vi "PointGrey Grasshopper_Cam.vi"(4 "Frames in sequence":u32, 6 "Image in":variant, 7 "Camera-specific in":variant, 8 "Save path":path, 9 "Capture mode":enum16{"Single frame", "Sequence"}(ring), 10 "Exposure time (s)":dbl, 11 "Operation":T2(ring)) -> (3 "Status":T1, 5 "Camera-specific out":variant)   [LabVIEW 2015]
uses:
  <vilib>/userdefined/High Color/IMAQdx.ctl
  <vilib>/vision/Image Controls.llb/IMAQ Image.ctl
  <vilib>/vision/driver/IMAQdx.llb/IMAQdx Camera Control Mode.ctl
  <vilib>/vision/driver/IMAQdx.llb/IMAQdx Buffer Number Mode.ctl
  <vilib>/vision/driver/NI_Vision_Acquisition_Software.lvlib
  <resource>/objmgr/imaqdx.rc
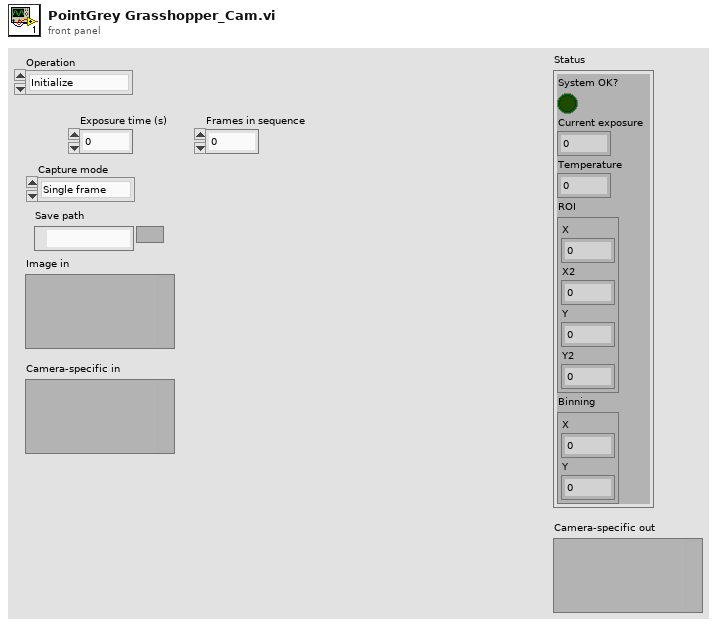
[diagram p1: front panel]
types:
  T1 = cluster{"System OK?":bool, "Current exposure":dbl, "Temperature":dbl, "ROI":cluster{"X":u32, "X2":u32, "Y":u32, "Y2":u32}, "Binning":cluster{"X":u32, "Y":u32}}
  T2 = enum16{"Initialize", "Shut down", "Set capture mode", "Set exposure", "Trigger and read", "Get status", "Other settings"}
  T3 = typedef "IMAQdx.ctl" = refnum<k21>
  T4 = typedef "IMAQ Image.ctl" = refnum<image>
  T5 = cluster{"Frames to capture":u32, "Current camera":i32, "Camera References":T3[], "Camera event refnum":refnum<event-registration>, "Which cameras record":bool[], "Image buffers":T4[]}
  T6 = enum32{"Continuous", "Single frame", "Multi frame"}
  T7 = typedef "NI_Vision_Acquisition_Software.lvlib/IMAQdx Camera Control Mode.ctl" = enum32{"Controller", "Listener"}
  T8 = cluster{"New Image":T4, "Image":refnum<vi>, "FPS target":dbl}
  T9 = enum16{"open", "replace", "create", "open or create", "replace or create", "replace or create with confirmation"}
  T10 = cluster{"File refnum":refnum<file>, "Image File Directory":cluster{cluster{"Field":u16, "Type":u16, "Count":u32, "Value / Offset":u32, "Add IFD Offset?":bool}[], cluster{"Data":u32[], "Add offset?":bool}[]}, "Big endian?":bool, "IFD Offset Size":u32}
  T11 = typedef "NI_Vision_Acquisition_Software.lvlib/IMAQdx Buffer Number Mode.ctl" = enum32{"Next", "Last", "Buffer Number", "Every", "Last New"}
  T12 = cluster{"Type":u32, "Version":u32, "Flags":u32, "SerialNumberHigh":u32, "SerialNumberLow":u32, "BusType":u32, "InterfaceName":string, "VendorName":string, "ModelName":string, "CameraFileName":string, "CameraAttributeURL":string}[]
  T13 = typedef "NI_Vision_Acquisition_Software.lvlib/IMAQdx Attribute Type.ctl" = enum32{"U32", "I64", "DBL", "String", "Enum", "Bool", "Command"}
  T14 = cluster{"Attribute Type":T13, "Readable":bool, "Writable":bool, "Attribute Name":string}[]
  T15 = typedef "Image Type" = u32
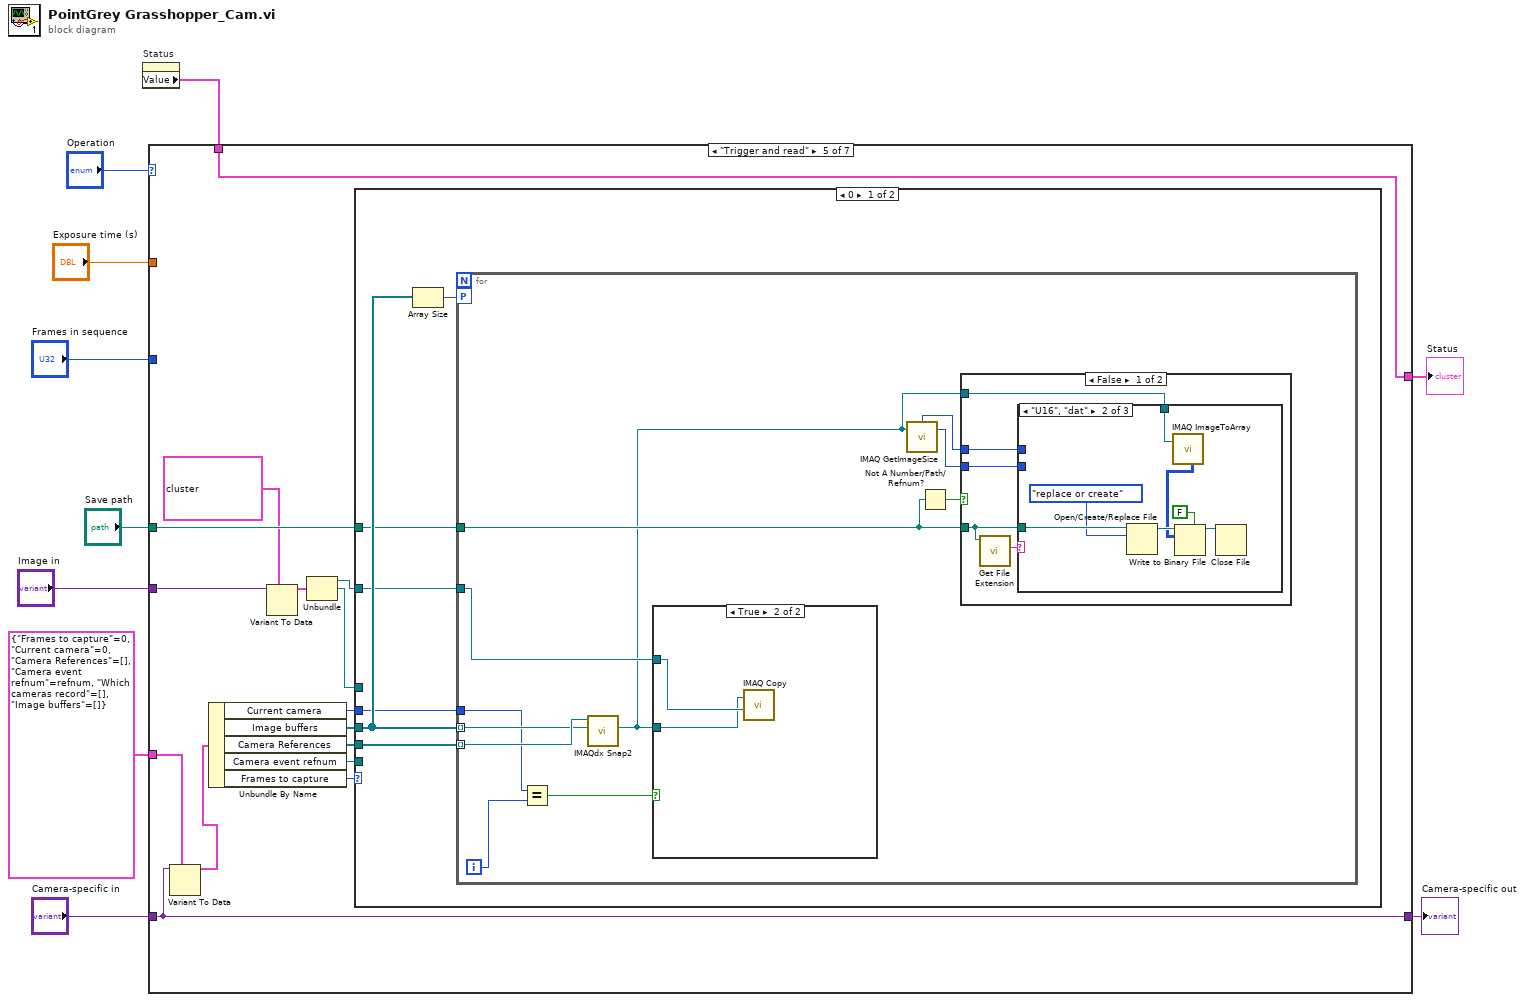
[diagram p0: block diagram]
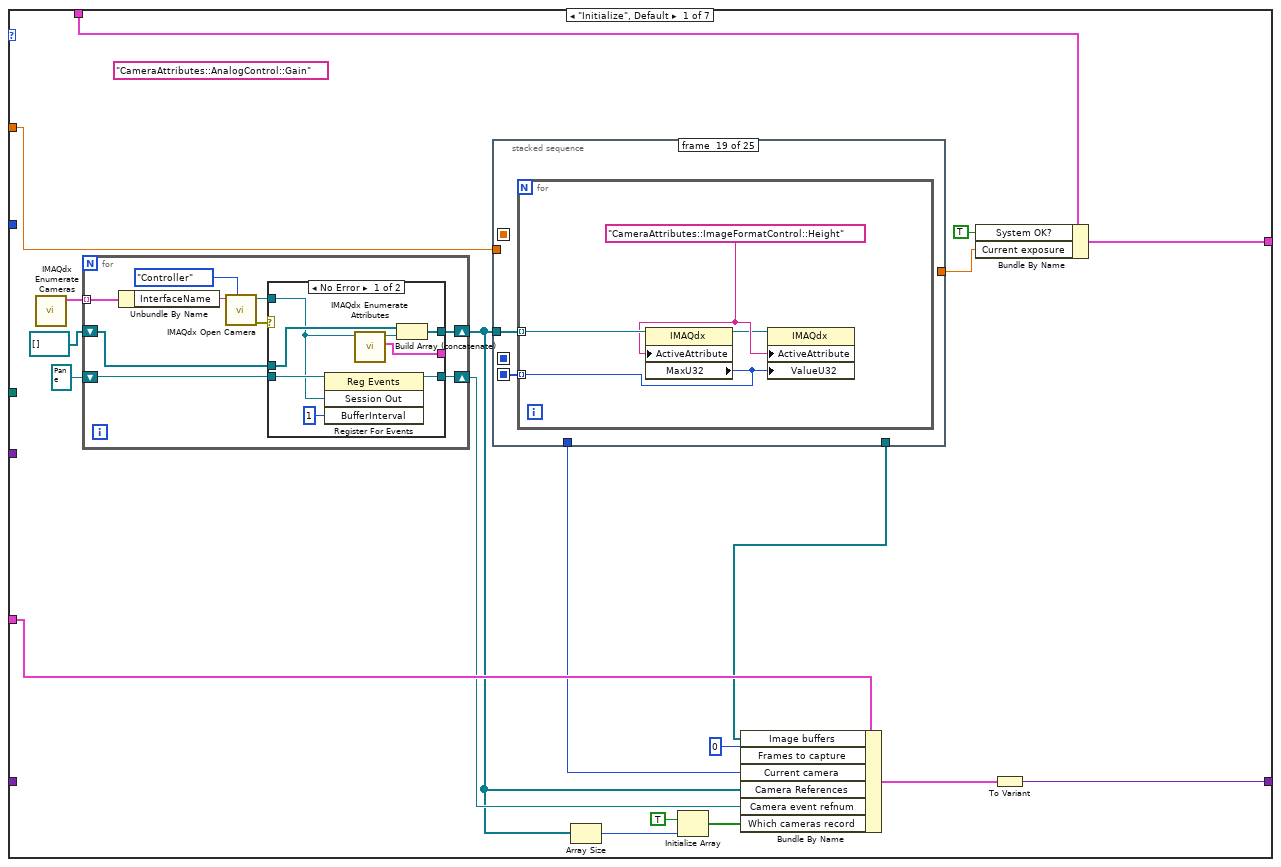
[diagram p2: hidden frame]
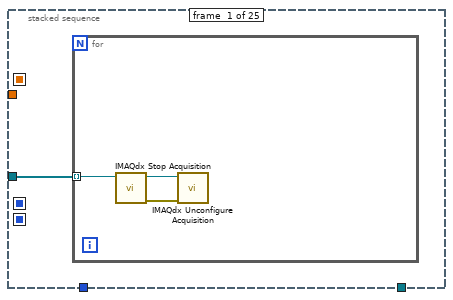
[diagram p3: hidden frame]
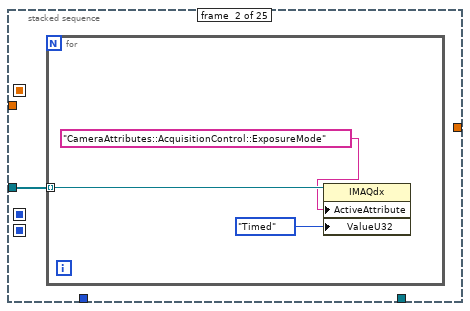
[diagram p4: hidden frame]
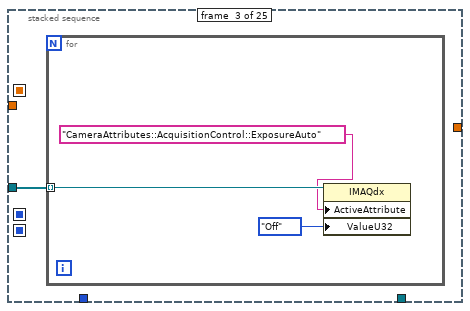
[diagram p5: hidden frame]
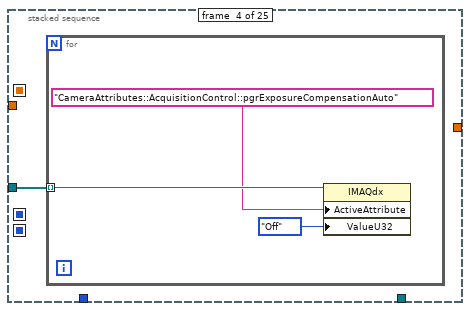
[diagram p6: hidden frame]
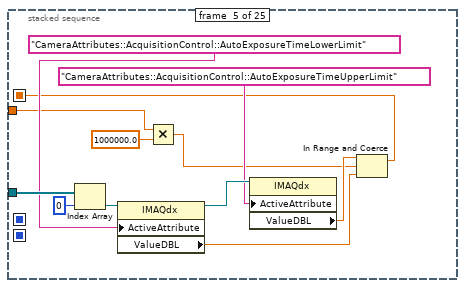
[diagram p7: hidden frame]
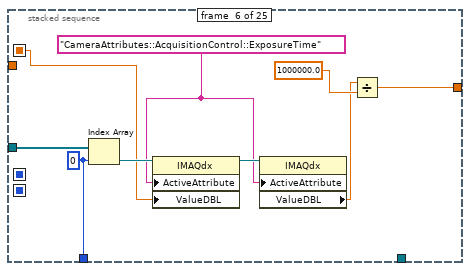
[diagram p8: hidden frame]
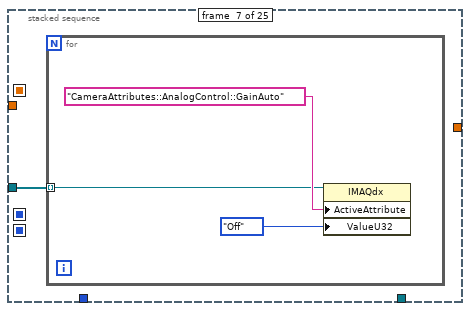
[diagram p9: hidden frame]
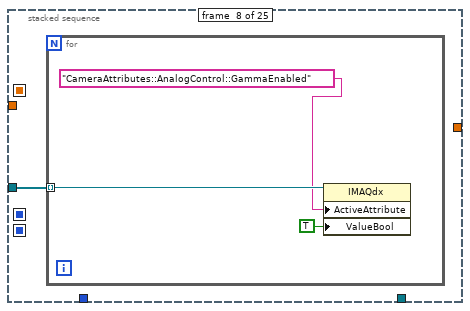
[diagram p10: hidden frame]
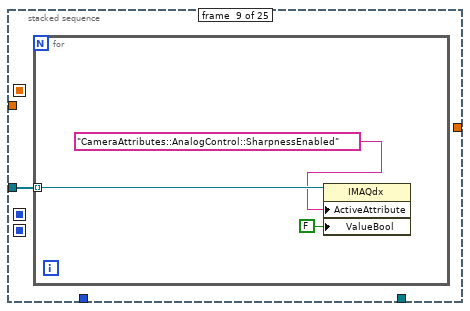
[diagram p11: hidden frame]
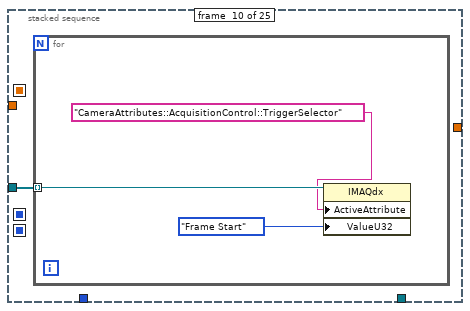
[diagram p12: hidden frame]
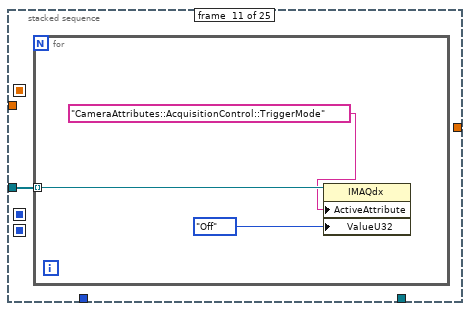
[diagram p13: hidden frame]
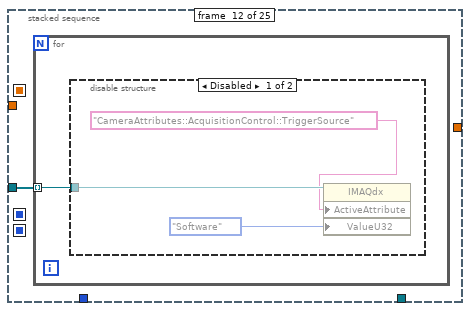
[diagram p14: hidden frame]
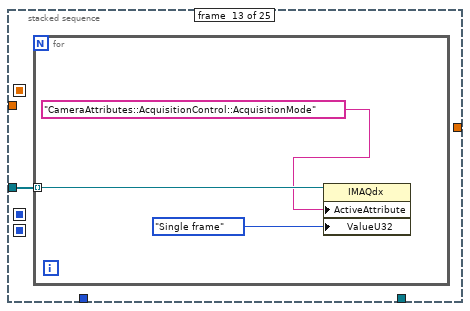
[diagram p16: hidden frame]
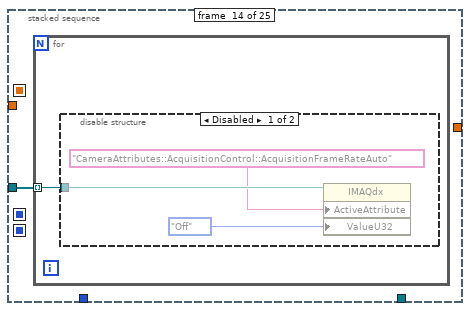
[diagram p17: hidden frame]
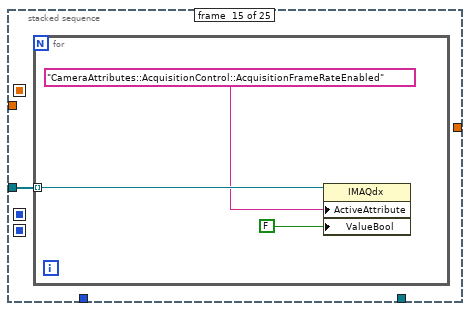
[diagram p19: hidden frame]
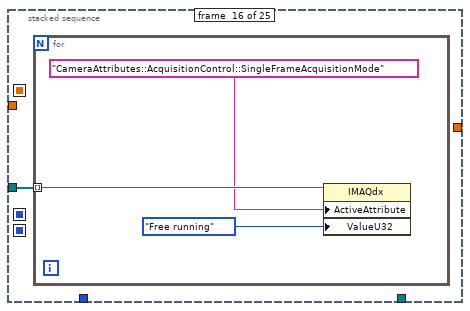
[diagram p20: hidden frame]
diagram:
  n1 = property on="Status" class="Clust (strict)"() -> ("Value"=w8:T1)  [unwired: 2 in, 2 out]
  n2 = case shown="\"Trigger and read\"" "Operation" {
    tunnel: "Exposure time (s)" -> [w17 _ _ w267 _ _ _]
    tunnel: w8 -> [w29 w183 w205 w273 w309 w509 w519]
    tunnel: [w28 w183 w205 w272 w309 w508 w519] -> w7
    tunnel: "Save path" -> [_ _ _ _ w308 _ _]
    tunnel: "Image in" -> [_ _ _ _ w297 _ _]
    tunnel: [w26 w178 w201 w270 w307 w505 w511] -> w4
    tunnel: "Camera-specific in" -> [_ w182 w203 w270 w307 w505 w518]
    tunnel: T5 {"Frames to capture"=0, "Current camera"=0, "Camera References"=[], "Camera event refnum"=refnum, "Which cameras record"=[], "Image buffers"=[]} -> [w27 w177 w202 w271 w306 w504 w517]
    tunnel: "Frames in sequence" -> [_ _ w198 _ _ _ _]
    frame "Initialize", Default {
      (unwired) "CameraAttributes::AnalogControl::Gain"
      n3 = call <vilib>:"IMAQdx Enumerate Cameras.vi"() -> ("Camera Information Array"=w24:T12)  [unwired: 10 in, 1 out]
      n4 = for {
        tunnel: w24 -> [w166] mode=indexing
        shift-right: [w162] -> w20
        shift-left: refnum<event-registration> refnum ("event registration refnum") -> [w161]
        shift-right: [w160] -> w15
        shift-left: T3[] [] -> [w158]
        n5 = Unbundle By Name(w166) -> ("InterfaceName"=w165:string)
        n6 = call <vilib>:"IMAQdx Open Camera.vi"("Camera Control Mode"=IMAQdx_Camera_Control_Mode."Controller", "Session In"=w165) -> ("error out"=w159:errorcluster, "Session Out"=w163:T3)  [unwired: 8 in]
        n7 = case shown="No Error" w159 {
          tunnel: w163 -> [w167 _]
          tunnel: [w173 w176] -> w162
          tunnel: w161 -> [w172 w176]
          tunnel: [w170 w175] -> w160
          tunnel: w158 -> [w169 w175]
          tunnel: [w168 _] -> _
          frame No Error {
            n8 = register-events(reference=w172, w167, u32 1 ("BufferInterval")) -> (reference out=w173:refnum<event-registration>)  [unwired: 1 in, 1 out]
            n9 = call <vilib>:"IMAQdx Enumerate Attributes.vi"("Session In"=w167) -> ("Attribute Information Array"=w168:T14, "Session Out"=w171:T3)  [unwired: 8 in, 1 out]
            n10 = Build Array (concatenate)(w169, w171) -> (w170:T3[])
          }
          frame Error {
          }
        }
      }
      n11 = stacked-sequence {
        seq-local: [_ _ _ _ w49 _ _ _ _ _ _ _ _ _ _ _ _ _ _ _ _ _ _ _ _] -> [_ _ _ _ _ w58 _ _ _ _ _ _ _ _ _ _ _ _ _ _ _ _ _ _ _]
        seq-local: [_ _ _ _ _ _ _ _ _ _ _ _ _ _ _ _ _ w113 _ _ _ _ _ _ _] -> [_ _ _ _ _ _ _ _ _ _ _ _ _ _ _ _ _ _ _ _ _ _ _ w143 _]
        seq-local: [_ _ _ _ _ _ _ _ _ _ _ _ _ _ _ _ _ _ w119 _ _ _ _ _ _] -> [_ _ _ _ _ _ _ _ _ _ _ _ _ _ _ _ _ _ _ _ _ _ _ w142 _]
        tunnel: w15 -> [w30 w34 w38 w42 w55 w65 w67 w71 w75 w79 w83 w87 w92 w96 w101 w105 w109 w114 w120 w125 w129 w133 w137 w144 w156]
        tunnel: [_ _ _ _ _ w64 _ _ _ _ _ _ _ _ _ _ _ _ _ _ _ _ _ _ _] -> w18
        tunnel: w17 -> [_ _ _ _ w47 _ _ _ _ _ _ _ _ _ _ _ _ _ _ _ _ _ _ _ _]
        tunnel: [_ _ _ _ _ w60 _ _ _ _ _ _ _ _ _ _ _ _ _ _ _ _ _ _ _] -> w16
        tunnel: [_ _ _ _ _ _ _ _ _ _ _ _ _ _ _ _ _ _ _ _ _ _ _ w141 _] -> w11
        frame #0 {
          n12 = for {
            tunnel: w30 -> [w33] mode=indexing
            n13 = call <vilib>:"IMAQdx Stop Acquisition.vi"("Session In"=w33) -> ("error out"=w31:errorcluster, "Session Out"=w32:T3)  [unwired: 9 in]
            n14 = call <vilib>:"IMAQdx Unconfigure Acquisition.vi"("error in"=w31, "Session In"=w32) -> ()  [unwired: 8 in, 2 out]
          }
        }
        frame #1 {
          n15 = for {
            tunnel: w34 -> [w37] mode=indexing
            n16 = property class="IMAQdx"(reference=w37, "ActiveAttribute"="CameraAttributes::AcquisitionControl::ExposureMode", "ValueU32"=enum32{"Timed", "Trigger Width"}."Timed") -> ()  [unwired: 1 in, 2 out]
          }
        }
        frame #2 {
          n17 = for {
            tunnel: w38 -> [w41] mode=indexing
            n18 = property class="IMAQdx"(reference=w41, "ActiveAttribute"="CameraAttributes::AcquisitionControl::ExposureAuto", "ValueU32"=enum32{"Off", "Once", "Continuous"}."Off") -> ()  [unwired: 1 in, 2 out]
          }
        }
        frame #3 {
          n19 = for {
            tunnel: w42 -> [w45] mode=indexing
            n20 = property class="IMAQdx"(reference=w45, "ActiveAttribute"="CameraAttributes::AcquisitionControl::pgrExposureCompensationAuto", "ValueU32"=enum32{"Off", "Once", "Continuous"}."Off") -> ()  [unwired: 1 in, 2 out]
          }
        }
        frame #4 {
          n21 = Index Array(array=w55, index=0) -> (element=w57:T3)
          n22 = property class="IMAQdx"(reference=w57, "ActiveAttribute"="CameraAttributes::AcquisitionControl::AutoExposureTimeLowerLimit") -> (reference out=w53:T3, "ValueDBL"=w51:dbl)  [unwired: 1 in, 1 out]
          n23 = Multiply(x=w47, y=1000000.0) -> (x*y=w46:dbl)
          n24 = property class="IMAQdx"(reference=w53, "ActiveAttribute"="CameraAttributes::AcquisitionControl::AutoExposureTimeUpperLimit") -> ("ValueDBL"=w50:dbl)  [unwired: 1 in, 2 out]
          n25 = In Range and Coerce(upper limit=w50, x=w46, lower limit=w51) -> (coerced(x)=w49:dbl)  [unwired: 1 out]
        }
        frame #5 {
          w59 = "CameraAttributes::AcquisitionControl::ExposureTime"
          w64 = 0 ("index")
          n26 = Index Array(array=w65, index=w64) -> (element=w66:T3)
          n27 = property class="IMAQdx"(reference=w66, "ActiveAttribute"=w59, "ValueDBL"=w58) -> (reference out=w63:T3)  [unwired: 1 in, 1 out]
          n28 = property class="IMAQdx"(reference=w63, "ActiveAttribute"=w59) -> ("ValueDBL"=w61:dbl)  [unwired: 1 in, 2 out]
          n29 = Divide(x=w61, y=1000000.0) -> (x/y=w60:dbl)
        }
        frame #6 {
          n30 = for {
            tunnel: w67 -> [w68] mode=indexing
            n31 = property class="IMAQdx"(reference=w68, "ActiveAttribute"="CameraAttributes::AnalogControl::GainAuto", "ValueU32"=enum32{"Off", "Once", "Continuous"}."Off") -> ()  [unwired: 1 in, 2 out]
          }
        }
        frame #7 {
          n32 = for {
            tunnel: w71 -> [w74] mode=indexing
            n33 = property class="IMAQdx"(reference=w74, "ActiveAttribute"="CameraAttributes::AnalogControl::GammaEnabled", "ValueBool"=TRUE) -> ()  [unwired: 1 in, 2 out]
          }
        }
        frame #8 {
          n34 = for {
            tunnel: w75 -> [w78] mode=indexing
            n35 = property class="IMAQdx"(reference=w78, "ActiveAttribute"="CameraAttributes::AnalogControl::SharpnessEnabled", "ValueBool"=FALSE) -> ()  [unwired: 1 in, 2 out]
          }
        }
        frame #9 {
          n36 = for {
            tunnel: w79 -> [w82] mode=indexing
            n37 = property class="IMAQdx"(reference=w82, "ActiveAttribute"="CameraAttributes::AcquisitionControl::TriggerSelector", "ValueU32"=enum32{"Frame Start", "Exposure Active"}."Frame Start") -> ()  [unwired: 1 in, 2 out]
          }
        }
        frame #10 {
          n38 = for {
            tunnel: w83 -> [w86] mode=indexing
            n39 = property class="IMAQdx"(reference=w86, "ActiveAttribute"="CameraAttributes::AcquisitionControl::TriggerMode", "ValueU32"=enum32{"Off", "On"}."Off") -> ()  [unwired: 1 in, 2 out]
          }
        }
        frame #11 {
          n40 = for {
            tunnel: w87 -> [w88] mode=indexing
            n41 = disable-structure shown="Disabled" {
              disable-tunnel: w88 -> [w91 _]
              frame Disabled {
                n42 = property class="IMAQdx"(reference=w91, "ActiveAttribute"="CameraAttributes::AcquisitionControl::TriggerSource", "ValueU32"=enum32{"Software", "Line 0", "Line 2", "Line 3"}."Software") -> ()  [unwired: 1 in, 2 out]
              }
              frame Enabled {
              }
            }
          }
        }
        frame #12 {
          n43 = for {
            tunnel: w92 -> [w95] mode=indexing
            n44 = property class="IMAQdx"(reference=w95, "ActiveAttribute"="CameraAttributes::AcquisitionControl::AcquisitionMode", "ValueU32"=T6."Single frame") -> ()  [unwired: 1 in, 2 out]
          }
        }
        frame #13 {
          n45 = for {
            tunnel: w96 -> [w97] mode=indexing
            n46 = disable-structure shown="Disabled" {
              disable-tunnel: w97 -> [w100 _]
              frame Disabled {
                n47 = property class="IMAQdx"(reference=w100, "ActiveAttribute"="CameraAttributes::AcquisitionControl::AcquisitionFrameRateAuto", "ValueU32"=enum32{"Off", "Continuous"}."Off") -> ()  [unwired: 1 in, 2 out]
              }
              frame Enabled {
              }
            }
          }
        }
        frame #14 {
          n48 = for {
            tunnel: w101 -> [w104] mode=indexing
            n49 = property class="IMAQdx"(reference=w104, "ActiveAttribute"="CameraAttributes::AcquisitionControl::AcquisitionFrameRateEnabled", "ValueBool"=FALSE) -> ()  [unwired: 1 in, 2 out]
          }
        }
        frame #15 {
          n50 = for {
            tunnel: w105 -> [w108] mode=indexing
            n51 = property class="IMAQdx"(reference=w108, "ActiveAttribute"="CameraAttributes::AcquisitionControl::SingleFrameAcquisitionMode", "ValueU32"=enum16{"Free running", "Triggered"}."Free running") -> ()  [unwired: 1 in, 2 out]
          }
        }
        frame #16 {
          n52 = for {
            tunnel: w109 -> [w112] mode=indexing
            w111 = u32 17563654 items=["Mono 8"=17301505, "Mono 12 Packed (IIDC-msb)"=17563654, "Mono 12 Packed"=17563719, "Mono 16"=17825799]
            n53 = property class="IMAQdx"(reference=w112, "ActiveAttribute"="CameraAttributes::ImageFormatControl::PixelFormat", "ValueU32"=w111) -> ()  [unwired: 1 in, 2 out]
          }
        }
        frame #17 {
          n54 = for {
            tunnel: w114 -> [w118] mode=indexing
            tunnel: [w115] -> w113 mode=indexing
            w117 = "CameraAttributes::ImageFormatControl::Width"
            n55 = property class="IMAQdx"(reference=w118, "ActiveAttribute"=w117) -> (reference out=w116:T3, "MaxU32"=w115:u32)  [unwired: 1 in, 1 out]
            n56 = property class="IMAQdx"(reference=w116, "ActiveAttribute"=w117, "ValueU32"=w115) -> ()  [unwired: 1 in, 2 out]
          }
        }
        frame #18 {
          n57 = for {
            tunnel: w120 -> [w124] mode=indexing
            tunnel: [w121] -> w119 mode=indexing
            w123 = "CameraAttributes::ImageFormatControl::Height"
            n58 = property class="IMAQdx"(reference=w124, "ActiveAttribute"=w123) -> (reference out=w122:T3, "MaxU32"=w121:u32)  [unwired: 1 in, 1 out]
            n59 = property class="IMAQdx"(reference=w122, "ActiveAttribute"=w123, "ValueU32"=w121) -> ()  [unwired: 1 in, 2 out]
          }
        }
        frame #19 {
          n60 = for {
            tunnel: w125 -> [w127] mode=indexing
            n61 = property class="IMAQdx"(reference=w127, "ActiveAttribute"="CameraAttributes::ImageFormatControl::OffsetX", "ValueU32"=u32 0) -> ()  [unwired: 1 in, 2 out]
          }
        }
        frame #20 {
          n62 = for {
            tunnel: w129 -> [w131] mode=indexing
            n63 = property class="IMAQdx"(reference=w131, "ActiveAttribute"="CameraAttributes::ImageFormatControl::OffsetY", "ValueU32"=u32 0) -> ()  [unwired: 1 in, 2 out]
          }
        }
        frame #21 {
          n64 = for {
            tunnel: w133 -> [w135] mode=indexing
            n65 = property class="IMAQdx"(reference=w135, "ActiveAttribute"="CameraAttributes::ImageFormatControl::BinningVertical", "ValueU32"=u32 1) -> ()  [unwired: 1 in, 2 out]
          }
        }
        frame #22 {
          n66 = for {
            tunnel: w137 -> [w139] mode=indexing
            w138 = u16 7 items=["Standard"=0, "2x2 Binning"=1, "2x2 Decimation"=2, "High sensitivity 12-bit ADC"=7]
            n67 = property class="IMAQdx"(reference=w139, "ActiveAttribute"="CameraAttributes::ImageFormatControl::VideoMode", "ValueU32"=w138) -> ()  [unwired: 1 in, 2 out]
          }
        }
        frame #23 {
          n68 = for {
            tunnel: w144 -> [_] mode=indexing
            tunnel: w143 -> [w148] mode=indexing
            tunnel: w142 -> [w147] mode=indexing
            tunnel: [w149] -> w141 mode=indexing
            i -> [w153]
            w155 = T15 7 items=["Grayscale (U8)", "Grayscale (I16)", "Grayscale (SGL)", "Complex (CSG)", "RGB (U32)", "HSL (U32)", "RGB (U64)", "Grayscale (U16)"] ("Image Type")
            n69 = Number To Decimal String(number=w153) -> (decimal integer string=w152:string)  [unwired: 1 in]
            n70 = Concatenate Strings("Image ", w152) -> (w151:string)
            n71 = call "IMAQ Create"("Image Name"=w151, "Image Type"=w155) -> ("New Image"=w150:T4)  [unwired: 3 in, 1 out]
            n72 = To Long Integer(number=w148) -> (32bit integer=w146:i32)
            n73 = To Long Integer(number=w147) -> (32bit integer=w145:i32)
            n74 = call "IMAQ SetImageSize"("Y Resolution"=w145, "X Resolution"=w146, "Image"=w150) -> ("Image Out"=w149:T4)  [unwired: 2 in, 1 out]
          }
        }
        frame #24 {
          n75 = for {
            tunnel: w156 -> [w157] mode=indexing
            n76 = call <vilib>:"IMAQdx Configure Grab.vi"("Session In"=w157) -> ()  [unwired: 9 in, 2 out]
          }
        }
      }
      n77 = Array Size(array=w15) -> (size(s)=w13:i32)
      n78 = Initialize Array(TRUE, w13) -> (w12:bool[])
      n79 = Bundle By Name(cluster=w27, "Image buffers"=w11, "Frames to capture"=u32 0, "Current camera"=w18, "Camera References"=w15, "Camera event refnum"=w20, "Which cameras record"=w12) -> (w21:T5)
      n80 = Bundle By Name(cluster=w29, "System OK?"=TRUE, "Current exposure"=w16) -> (w28:T1)
      n81 = To Variant(anything=w21) -> (Variant=w26:variant)
    }
    frame "Shut down" {
      n82 = Variant To Data(type=w177, Variant=w182) -> (data=w181:T5)  [unwired: 1 in, 1 out]
      n83 = Unbundle By Name(w181) -> ("Camera References"=w180:T3[], "Camera event refnum"=w179:refnum<event-registration>)
      n84 = stacked-sequence {
        tunnel: w180 -> [w184 _]
        tunnel: w179 -> [_ w191]
        frame #0 {
          n85 = for {
            tunnel: w184 -> [w185] mode=indexing
            n86 = call <vilib>:"IMAQdx Stop Acquisition.vi"("Session In"=w185) -> ("error out"=w189:errorcluster, "Session Out"=w188:T3)  [unwired: 9 in]
            n87 = call <vilib>:"IMAQdx Unconfigure Acquisition.vi"("error in"=w189, "Session In"=w188) -> ("error out"=w187:errorcluster, "Session Out"=w186:T3)  [unwired: 8 in]
            n88 = call <vilib>:"IMAQdx Close Camera.vi"("error in"=w187, "Session In"=w186) -> ()  [unwired: 9 in, 1 out]
          }
        }
        frame #1 {
          n89 = Unregister For Events(event registration refnum=w191) -> (error out=w190:errorcluster)  [unwired: 1 in]
          n90 = call <vilib>:"Clear Errors.vi"("error in (no error)"=w190) -> ()  [unwired: 5 in, 2 out]
        }
      }
      n91 = To Variant(anything=w177) -> (Variant=w178:variant)
    }
    frame "Set capture mode" {
      n92 = Variant To Data(type=w202, Variant=w203) -> (data=w197:T5)  [unwired: 1 in, 1 out]
      n93 = Unbundle By Name(w197) -> ("Camera References"=w196:T3[], "Camera event refnum"=w194:refnum<event-registration>, "Which cameras record"=w195:bool[])
      n94 = case shown="\"Single frame\", Default" "Capture mode" {
        tunnel: [u32 0 ("Frames in sequence") w208] -> w199
        tunnel: w198 -> [_ w209]
        tunnel: w196 -> [_ w214]
        tunnel: w195 -> [_ w213]
        tunnel: w194 -> [w207 w212]
        tunnel: [w207 w210] -> w193
        tunnel: refnum<event-registration> refnum ("Camera event refnum") -> [_ w211]
        frame "Single frame", Default {
          # "TEMPORARY"
        }
        frame "Sequence" {
          n95 = stacked-sequence {
            tunnel: w214 -> [_ w221]
            tunnel: w213 -> [_ w220]
            tunnel: w212 -> [w216 _]
            tunnel: w211 -> [_ w219]
            tunnel: [_ w218] -> w210
            tunnel: w209 -> [w215 w217]
            tunnel: [w215 _] -> w208
            frame #0 {
              n96 = Unregister For Events(event registration refnum=w216) -> ()  [unwired: 1 in, 1 out]
            }
            frame #1 {
              n97 = for {
                tunnel: w221 -> [w225] mode=indexing
                tunnel: w220 -> [w226] mode=indexing
                shift-right: [w224] -> w218
                shift-left: w219 -> [w223]
                tunnel: w217 -> [w222]
                n98 = case shown="True" w226 {
                  tunnel: w225 -> [_ w229]
                  tunnel: [w227 w230] -> w224
                  tunnel: w223 -> [w227 w231]
                  tunnel: w222 -> [_ w228]
                  frame False {
                  }
                  frame True {
                    n99 = stacked-sequence {
                      tunnel: w231 -> [_ w238 _ _ _ _ _ _ _]
                      tunnel: [_ w237 _ _ _ _ _ _ _] -> w230
                      tunnel: w229 -> [w234 w236 w239 w247 w251 w254 w258 w260 w263]
                      tunnel: w228 -> [_ _ _ w246 _ _ _ _ _]
                      frame #0 {
                        n100 = call <vilib>:"IMAQdx Stop Acquisition.vi"("Session In"=w234) -> ("error out"=w232:errorcluster, "Session Out"=w233:T3)  [unwired: 9 in]
                        n101 = call <vilib>:"IMAQdx Unconfigure Acquisition.vi"("error in"=w232, "Session In"=w233) -> ()  [unwired: 8 in, 2 out]
                      }
                      frame #1 {
                        n102 = register-events(reference=w238, w236, u32 1 ("BufferInterval")) -> (reference out=w237:refnum<event-registration>)  [unwired: 1 in, 1 out]
                      }
                      frame #2 {
                        n103 = disable-structure shown="Disabled" {
                          disable-tunnel: w239 -> [w240 w243]
                          frame Disabled {
                            n104 = property class="IMAQdx"(reference=w240, "ActiveAttribute"="CameraAttributes::AcquisitionControl::AcquisitionMode", "ValueU32"=T6."Multi frame") -> ()  [unwired: 1 in, 2 out]
                          }
                          frame Enabled {
                            n105 = property class="IMAQdx"(reference=w243, "ActiveAttribute"="CameraAttributes::AcquisitionControl::AcquisitionMode", "ValueU32"=T6."Continuous") -> ()  [unwired: 1 in, 2 out]
                          }
                        }
                      }
                      frame #3 {
                        n106 = disable-structure shown="Disabled" {
                          disable-tunnel: w247 -> [w249 _]
                          disable-tunnel: w246 -> [w248 _]
                          frame Disabled {
                            n107 = property class="IMAQdx"(reference=w249, "ActiveAttribute"="CameraAttributes::AcquisitionControl::AcquisitionFrameCount", "ValueU32"=w248) -> ()  [unwired: 1 in, 2 out]
                          }
                          frame Enabled {
                          }
                        }
                      }
                      frame #4 {
                        n108 = property class="IMAQdx"(reference=w251, "ActiveAttribute"="CameraAttributes::AcquisitionControl::TriggerSource", "ValueU32"=enum32{"Software", "Line 0", "Line 2", "Line 3"}."Software") -> ()  [unwired: 1 in, 2 out]
                      }
                      frame #5 {
                        n109 = property class="IMAQdx"(reference=w254, "ActiveAttribute"="CameraAttributes::AcquisitionControl::TriggerSelector", "ValueU32"=enum32{"Frame Start", "Exposure Active"}."Frame Start") -> ()  [unwired: 1 in, 2 out]
                      }
                      frame #6 {
                        n110 = property class="IMAQdx"(reference=w258, "ActiveAttribute"="CameraAttributes::AcquisitionControl::TriggerMode", "ValueU32"=enum32{"Off", "On"}."Off") -> ()  [unwired: 1 in, 2 out]
                      }
                      frame #7 {
                        n111 = property class="IMAQdx"(reference=w260, "ActiveAttribute"="CameraAttributes::AcquisitionControl::SingleFrameAcquisitionMode", "ValueU32"=enum16{"Free running", "Triggered"}."Triggered") -> ()  [unwired: 1 in, 2 out]
                      }
                      frame #8 {
                        n112 = disable-structure shown="Disabled" {
                          disable-tunnel: w263 -> [w264 _]
                          frame Disabled {
                            n113 = call <vilib>:"IMAQdx Configure Grab.vi"("Session In"=w264) -> ()  [unwired: 9 in, 2 out]
                          }
                          frame Enabled {
                          }
                        }
                      }
                    }
                  }
                }
              }
            }
          }
        }
      }
      n114 = Bundle By Name(cluster=w197, "Frames to capture"=w199, "Camera event refnum"=w193) -> (w200:T5)
      n115 = To Variant(anything=w200) -> (Variant=w201:variant)
    }
    frame "Set exposure" {
      n116 = Variant To Data(type=w271, Variant=w270) -> (data=w269:T5)  [unwired: 1 in, 1 out]
      n117 = Unbundle By Name(w269) -> ("Camera References"=w266:T3[], "Current camera"=w265:i32)
      n118 = stacked-sequence {
        seq-local: [w278 _] -> [_ w287]
        tunnel: w266 -> [w284 w293]
        tunnel: w267 -> [w276 _]
        tunnel: [_ w289] -> w268
        tunnel: w265 -> [w274 w286]
        frame #0 {
          n119 = Index Array(array=w284, index=w274) -> (element=w285:T3)
          n120 = property class="IMAQdx"(reference=w285, "ActiveAttribute"="CameraAttributes::AcquisitionControl::AutoExposureTimeLowerLimit") -> (reference out=w282:T3, "ValueDBL"=w280:dbl)  [unwired: 1 in, 1 out]
          n121 = Multiply(x=w276, y=1000000.0) -> (x*y=w275:dbl)
          n122 = property class="IMAQdx"(reference=w282, "ActiveAttribute"="CameraAttributes::AcquisitionControl::AutoExposureTimeUpperLimit") -> ("ValueDBL"=w279:dbl)  [unwired: 1 in, 2 out]
          n123 = In Range and Coerce(upper limit=w279, x=w275, lower limit=w280) -> (coerced(x)=w278:dbl)  [unwired: 1 out]
        }
        frame #1 {
          w288 = "CameraAttributes::AcquisitionControl::ExposureTime"
          n124 = Index Array(array=w293, index=w286) -> (element=w294:T3)
          n125 = property class="IMAQdx"(reference=w294, "ActiveAttribute"=w288, "ValueDBL"=w287) -> (reference out=w292:T3)  [unwired: 1 in, 1 out]
          n126 = property class="IMAQdx"(reference=w292, "ActiveAttribute"=w288) -> ("ValueDBL"=w290:dbl)  [unwired: 1 in, 2 out]
          n127 = Divide(x=w290, y=1000000.0) -> (x/y=w289:dbl)
        }
      }
      n128 = Bundle By Name(cluster=w273, "Current exposure"=w268) -> (w272:T1)
    }
    frame "Trigger and read" {
      n129 = Variant To Data(type=w306, Variant=w307) -> (data=w304:T5)  [unwired: 1 in, 1 out]
      n130 = Unbundle By Name(w304) -> ("Current camera"=w300:i32, "Image buffers"=w301:T4[], "Camera References"=w303:T3[], "Camera event refnum"=w302:refnum<event-registration>, "Frames to capture"=w305:u32)
      n131 = Variant To Data(type=T8 {"New Image"=refnum, "Image"=refnum, "FPS target"=30.0} ("output cluster"), Variant=w297) -> (data=w299:T8)  [unwired: 1 in, 1 out]
      n132 = Unbundle(w299) -> ("New Image"=w296:T4, "Image"=w295:refnum<vi>)  [unwired: 1 out]
      n133 = case shown="0" w305 {
        selector: w305 -> [_ w357]
        tunnel: w308 -> [w310 w363]
        tunnel: w296 -> [w311 w362]
        tunnel: w303 -> [w315 w361]
        tunnel: w302 -> [_ w360]
        tunnel: w301 -> [w313 w359]
        tunnel: w300 -> [w312 w358]
        tunnel: w295 -> [_ w356]
        frame 0 {
          n134 = Array Size(array=w313) -> (size(s)=w314:i32)
          n135 = for {
            tunnel: w313 -> [w325] mode=indexing
            tunnel: w315 -> [w326] mode=indexing
            workers-P: w314 -> [_]
            tunnel: w312 -> [w324]
            tunnel: w311 -> [w321]
            tunnel: w310 -> [w317]
            i -> [w323]
            n136 = Equal?(x=w324, y=w323) -> (x = y?=w322:bool)
            n137 = call <vilib>:"IMAQdx Snap2.vi"("Image In"=w325, "Session In"=w326) -> ("Image Out"=w316:T4)  [unwired: 7 in, 2 out]
            n138 = case shown="True" w322 {
              tunnel: w316 -> [_ w354]
              tunnel: w321 -> [_ w355]
              frame False {
              }
              frame True {
                n139 = call "IMAQ Copy"("Image Dst"=w355, "Image Src"=w354) -> ()  [unwired: 4 in, 2 out]
              }
            }
            n140 = call "IMAQ GetImageSize"("Image"=w316) -> ("Y Resolution"=w318:i32, "X Resolution"=w319:i32)  [unwired: 3 in, 1 out]
            n141 = Not A Number/Path/Refnum?(number/path/refnum=w317) -> (NaN/Path/Refnum?=w320:bool)
            n142 = case shown="False" w320 {
              tunnel: w317 -> [w330 _]
              tunnel: w316 -> [w331 _]
              tunnel: w319 -> [w328 _]
              tunnel: w318 -> [w327 _]
              frame False {
                n143 = call <vilib>:"Get File Extension.vi"("file"=w330) -> ("lowercase file extension"=w329:string)  [unwired: 6 in, 4 out]
                n144 = case shown="\"U16\", \"dat\"" w329 {
                  tunnel: w330 -> [w344 w353 _]
                  tunnel: w331 -> [w334 w348 _]
                  tunnel: w328 -> [w342 _ _]
                  tunnel: w327 -> [w341 _ _]
                  frame "'tiff'", "tif" {
                    n145 = call "TIFFStream Open.vi"("Bytes per strip"=u32 8000, "File path"=w344, "Height Pixels"=w341, "Width Pixels"=w342, "Big endian?"=FALSE) -> ("error out"=w338:errorcluster, "Next IFD Offset"=w336:u32, "Image data reference"=w335:refnum<data-value>, "File data"=w340:T10)  [unwired: 3 in]
                    n146 = in-place {
                      in-place-border: w334 -> [w346]
                      n147 = in-place-dvr #1(w335) -> ()  [unwired: 2 out]
                      n148 = call "IMAQ ImageToArray"("Image"=w346) -> ("Image Pixels (U16)"=w345:u16[][])  [unwired: 3 in, 4 out]
                      n149 = in-place-dvr #1(w345) -> (w332:refnum<data-value>)  [unwired: 1 out]
                    }
                    n150 = call "TIFFStream Write.vi"("File data"=w340, "error in (no error)"=w338, "Last image in file?"=TRUE, "IFD Offset"=w336, "Image data reference"=w332) -> ("error out"=w339:errorcluster)  [unwired: 5 in, 1 out]
                    n151 = call "TIFFStream Close.vi"("error in (no error)"=w339, "Image data reference"=w332, "File data"=w340) -> ()  [unwired: 8 in, 1 out]
                  }
                  frame "U16", "dat" {
                    n152 = Open/Create/Replace File(file path (use dialog)=w353, operation (0:open)=T9."replace or create") -> (refnum out=w352:refnum<file>)  [unwired: 4 in, 2 out]
                    n153 = call "IMAQ ImageToArray"("Image"=w348) -> ("Image Pixels (U16)"=w347:u16[][])  [unwired: 3 in, 4 out]
                    n154 = Write to Binary File(file (use dialog)=w352, data=w347, 5:FALSE ("prepend array or string size? (T)")) -> (refnum out=w350:refnum<file>)  [unwired: 3 in, 2 out]
                    n155 = Close File(refnum=w350) -> ()  [unwired: 1 in, 2 out]
                  }
                  frame "None", Default {
                  }
                }
              }
              frame True {
              }
            }
          }
        }
        frame 1, Default {
          n156 = stacked-sequence {
            seq-local: [w375 _ _] -> [_ w418 w491]
            seq-local: [w374 _ _] -> [_ w419 w490]
            seq-local: [w373 _ _] -> [_ w417 w489]
            seq-local: [w372 _ _] -> [_ w416 w488]
            seq-local: [w371 _ _] -> [_ w415 _]
            tunnel: w363 -> [w377 w429 _]
            tunnel: w362 -> [_ w428 _]
            tunnel: w361 -> [w368 w424 w492]
            tunnel: w360 -> [_ w427 _]
            tunnel: w359 -> [_ w426 _]
            tunnel: w358 -> [_ w425 _]
            tunnel: w357 -> [_ w421 _]
            tunnel: w356 -> [_ w414 _]
            frame #0 {
              # "Start acquisition"
              n157 = for {
                tunnel: w368 -> [w410] mode=indexing
                n158 = disable-structure shown="Disabled" {
                  disable-tunnel: w410 -> [w412 w413]
                  frame Disabled {
                    n159 = property class="IMAQdx"(reference=w412, "ActiveAttribute"="CameraAttributes::AcquisitionControl::TriggerSoftware") -> ()  [unwired: 1 in, 2 out]
                  }
                  frame Enabled {
                    n160 = call <vilib>:"IMAQdx Configure Grab.vi"("Session In"=w413) -> ()  [unwired: 9 in, 2 out]
                  }
                }
              }
              n161 = Index Array(array=w368, index=0) -> (element=w366:T3)
              n162 = property class="IMAQdx"(reference=w366, "ActiveAttribute"="CameraAttributes::ImageFormatControl::Width") -> ("ValueU32"=w369:u32)  [unwired: 1 in, 2 out]
              n163 = property class="IMAQdx"(reference=w366, "ActiveAttribute"="CameraAttributes::ImageFormatControl::Height") -> ("ValueU32"=w364:u32)  [unwired: 1 in, 2 out]
              n164 = Not A Number/Path/Refnum?(number/path/refnum=w377) -> (NaN/Path/Refnum?=w376:bool)
              n165 = case shown="False" w376 {
                tunnel: w377 -> [w385 _]
                tunnel: w369 -> [w384 _]
                tunnel: w364 -> [w383 _]
                tunnel: [w382 T10 {"File refnum"=refnum, "Image File Directory"={[], []}, "Big endian?"=FALSE, "IFD Offset Size"=0} ("File data")] -> w373
                tunnel: [w381 refnum<data-value> refnum ("Image data reference")] -> w372
                tunnel: [w380 u32 0 ("Next IFD Offset")] -> w371
                tunnel: [w379 refnum<file> refnum ("refnum out")] -> w374
                tunnel: [w378 "None" ("lowercase file extension")] -> w375
                frame False {
                  n166 = call <vilib>:"Get File Extension.vi"("file"=w385) -> ("lowercase file extension"=w378:string)  [unwired: 6 in, 4 out]
                  n167 = case shown="\"U16\", \"dat\"" w378 {
                    tunnel: w385 -> [w394 w400 _]
                    tunnel: w384 -> [w392 _ _]
                    tunnel: w383 -> [w391 _ _]
                    tunnel: [w389 T10 {"File refnum"=refnum, "Image File Directory"={[], []}, "Big endian?"=FALSE, "IFD Offset Size"=0} ("File data") T10 {"File refnum"=refnum, "Image File Directory"={[], []}, "Big endian?"=FALSE, "IFD Offset Size"=0} ("File data")] -> w382
                    tunnel: [w388 refnum<data-value> refnum ("Image data reference") refnum<data-value> refnum ("Image data reference")] -> w381
                    tunnel: [w387 u32 0 ("Next IFD Offset") u32 0 ("Next IFD Offset")] -> w380
                    tunnel: [refnum<file> refnum ("refnum out") w398 refnum<file> refnum ("refnum out")] -> w379
                    frame "'tiff'", "tif" {
                      n168 = call "TIFFStream Open.vi"("Bytes per strip"=u32 8000, "File path"=w394, "Height Pixels"=w391, "Width Pixels"=w392, "Big endian?"=FALSE) -> ("Next IFD Offset"=w387:u32, "Image data reference"=w388:refnum<data-value>, "File data"=w389:T10)  [unwired: 3 in, 1 out]
                    }
                    frame "U16", "dat" {
                      n169 = Open/Create/Replace File(file path (use dialog)=w400, operation (0:open)=T9."replace or create") -> (refnum out=w398:refnum<file>)  [unwired: 4 in, 2 out]
                    }
                    frame "None ", Default {
                    }
                  }
                }
                frame True {
                }
              }
            }
            frame #1 {
              n170 = To Long Integer(number=w421) -> (32bit integer=w420:i32)
              n171 = Array Size(array=w424) -> (size(s)=w423:i32)
              n172 = Multiply(x=w423, y=w420) -> (x*y=w422:i32)
              n173 = for {
                N: w422 -> [_]
                tunnel: w429 -> [w441]
                tunnel: w428 -> [w440]
                tunnel: w427 -> [w439]
                tunnel: w424 -> [w438]
                tunnel: w426 -> [w437]
                tunnel: w425 -> [w436]
                tunnel: w419 -> [w434]
                tunnel: w418 -> [w433]
                tunnel: w417 -> [w432]
                tunnel: w416 -> [w431]
                border: w415 -> [_]
                tunnel: w414 -> [w430]
                n174 = event shown="[1] <Session Out>: Frame Done" {
                  selector: w439 -> [_ _]
                  dyn-events: _ -> [_ _]
                  timeout: 1000 -> [_ _]
                  tunnel: w441 -> [_ _]
                  tunnel: w440 -> [_ w458]
                  tunnel: w438 -> [_ w456]
                  tunnel: w437 -> [_ w455]
                  tunnel: w436 -> [_ w452]
                  tunnel: w434 -> [_ w446]
                  tunnel: w433 -> [_ w445]
                  tunnel: w432 -> [_ w444]
                  tunnel: w431 -> [_ w443]
                  tunnel: w430 -> [_ w442]
                  event Timeout {
                    n175 = event-data() -> ()  [unwired: 1 in, 2 out]
                  }
                  event event #0x0 {
                    (unwired) FALSE ("Wait for Next Buffer? (Yes)")
                    # "Read data"
                    n176 = event-data() -> ("CtlRef"=w457:T3)  [unwired: 1 in, 3 out]
                    n177 = Not A Number/Path/Refnum?(number/path/refnum=w458) -> (NaN/Path/Refnum?=w459:bool)
                    n178 = property class="IMAQdx"(reference=w457) -> ("SerialNumberLow"=w454:u32)  [unwired: 1 in, 2 out]
                    n179 = for {
                      tunnel: w456 -> [w479] mode=indexing
                      tunnel: w455 -> [w477] mode=indexing
                      tunnel: [w478] -> w449
                      tunnel: [w477] -> w450
                      tunnel: w454 -> [w475]
                      tunnel: [w473] -> w453
                      i -> [w473]
                      stop <- w474 stop-if-true
                      n180 = property class="IMAQdx"(reference=w479) -> (reference out=w478:T3, "SerialNumberLow"=w476:u32)  [unwired: 1 in, 1 out]
                      n181 = Equal?(x=w475, y=w476) -> (x = y?=w474:bool)
                    }
                    n182 = Equal?(x=w453, y=w452) -> (x = y?=w451:bool)
                    n183 = call <vilib>:"IMAQdx Get Image2.vi"("Buffer Number Mode (Next)"=IMAQdx_Buffer_Number_Mode."Last New", "Image In"=w450, "Session In"=w449) -> ("Image Out"=w447:T4)  [unwired: 5 in, 3 out]
                    n184 = case shown="False" w459 {
                      tunnel: w458 -> [w482 _]
                      tunnel: w451 -> [w483 _]
                      tunnel: w447 -> [w481 _]
                      tunnel: w442 -> [w480 _]
                      frame False {
                        n185 = case shown="True" w483 {
                          tunnel: w482 -> [_ w487]
                          tunnel: w481 -> [_ w486]
                          tunnel: w480 -> [_ w485]
                          frame False {
                          }
                          frame True {
                            n186 = call "IMAQ Copy"("Image Dst"=w487, "Image Src"=w486) -> ("Image Dst Out"=w484:T4)  [unwired: 4 in, 1 out]
                            n187 = property class="ImageControl"(reference=w485, "Value"=w484) -> ()  [unwired: 1 in, 2 out]
                          }
                        }
                      }
                      frame True {
                      }
                    }
                    n188 = case shown="\"U16\", \"dat\"" w445 {
                      tunnel: w450 -> [w465 _ w471]
                      tunnel: w446 -> [_ _ w469]
                      tunnel: w444 -> [w462 _ _]
                      tunnel: w443 -> [w463 _ _]
                      frame "'tiff'", "tif" {
                        n189 = in-place {
                          in-place-border: w465 -> [w468]
                          n190 = in-place-dvr #2(w463) -> ()  [unwired: 2 out]
                          n191 = call "IMAQ ImageToArray"("Image"=w468) -> ("Image Pixels (U16)"=w467:u16[][])  [unwired: 3 in, 4 out]
                          n192 = in-place-dvr #2(w467) -> (w464:refnum<data-value>)  [unwired: 1 out]
                        }
                        n193 = feedback #3() -> (w461:u32)
                        n194 = call "TIFFStream Write.vi"("File data"=w462, "Last image in file?"=TRUE, "IFD Offset"=w461, "Image data reference"=w464) -> ("Next IFD Offset"=w460:u32)  [unwired: 6 in, 1 out]
                        n195 = feedback-in #3(w460) -> ()
                      }
                      frame "None", Default {
                      }
                      frame "U16", "dat" {
                        n196 = call "IMAQ ImageToArray"("Image"=w471) -> ("Image Pixels (U16)"=w470:u16[][])  [unwired: 3 in, 4 out]
                        n197 = Write to Binary File(file (use dialog)=w469, data=w470, 5:FALSE ("prepend array or string size? (T)")) -> ()  [unwired: 3 in, 3 out]
                      }
                    }
                  }
                }
              }
            }
            frame #2 {
              n198 = disable-structure shown="Enabled" {
                disable-tunnel: w492 -> [_ w496]
                frame Disabled {
                }
                frame Enabled {
                  n199 = for {
                    tunnel: w496 -> [w497] mode=indexing
                    n200 = call <vilib>:"IMAQdx Stop Acquisition.vi"("Session In"=w497) -> ()  [unwired: 9 in, 2 out]
                  }
                }
              }
              n201 = case shown="\"None\", Default" w491 {
                tunnel: w490 -> [_ _ w495]
                tunnel: w489 -> [w494 _ _]
                tunnel: w488 -> [w493 _ _]
                frame "'tiff'", "tif" {
                  n202 = call "TIFFStream Close.vi"("Image data reference"=w493, "File data"=w494) -> ()  [unwired: 9 in, 1 out]
                }
                frame "None", Default {
                }
                frame "U16", "dat" {
                  n203 = Close File(refnum=w495) -> ()  [unwired: 1 in, 2 out]
                }
              }
            }
          }
        }
      }
    }
    frame "Get status" {
      n204 = Variant To Data(type=w504, Variant=w505) -> (data=w503:T5)  [unwired: 1 in, 1 out]
      n205 = Unbundle By Name(w503) -> ("Camera References"=w502:T3[], "Current camera"=w501:i32)
      n206 = Index Array(array=w502, index=w501) -> (element=w500:T3)
      n207 = property class="IMAQdx"(reference=w500, "ActiveAttribute"="CameraAttributes::DeviceControl::DeviceTemperature") -> (error out=w499:errorcluster, "ValueDBL"=w506:dbl)  [unwired: 1 in, 1 out]
      n208 = Unbundle By Name(w499) -> ("status"=w498:bool)
      n209 = Bundle By Name(cluster=w509, "System OK?"=w498, "Temperature"=w506) -> (w508:T1)
    }
    frame "Other settings" {
      n210 = Variant To Data(type=w517, Variant=w518) -> (data=w513:T5)  [unwired: 1 in, 1 out]
      n211 = Unbundle By Name(w513) -> ("Camera References"=w516:T3[], "Current camera"=w515:i32, "Which cameras record"=w514:bool[])
      n212 = call "PointGrey Grasshopper_Settings.vi"("Which cameras record"=w514, "Camera to address"=w515, "Camera References"=w516) -> ("Which cameras record out"=w512:bool[])  [unwired: 8 in]
      n213 = Bundle By Name(cluster=w513, "Which cameras record"=w512) -> (w510:T5)
      n214 = To Variant(anything=w510) -> (Variant=w511:variant)
    }
  }
  "Status" <- w7
  "Camera-specific out" <- w4
